vi "Actor Core.vi"(8 "error in":errorcluster, 11 "Square in":refnum<class "Rigol DG822 Pulse.lvclass">) -> (0 "error out":errorcluster, 3 "Actor out":refnum<class "Actor.lvclass">)   [LabVIEW 2021, in "Rigol DG822 UI.lvlib" / "Rigol DG822 Pulse.lvlib" / "Rigol DG822 Pulse.lvclass"]
uses:
  Rigol DG822 Pulse.lvclass
  D:/LabVIEW/General/Files/lvlibp/Actors.lvlibp/Actors/Actors/Actors.lvclass
  General/Files/lvlibp/Actor Framework.lvlibp/1abvi3w/vi.lib/ActorFramework/Actor/Actor.lvclass
  Rigol DG822 UI/lib/controls.llb/FreqUnitHandler.ctl
  Rigol DG822 UI/lib/controls.llb/DataCluster.ctl
  Rigol DG822 UI/lib/controls.llb/PeriodUnitHandler.ctl
  Rigol DG822 UI/lib/controls.llb/AmplUnitHandler.ctl
  Rigol DG822 UI/lib/controls.llb/HighLUnitHandler.ctl
  Rigol DG822 UI/lib/controls.llb/OffsetUnitHandler.ctl
  Rigol DG822 UI/lib/controls.llb/LowLUnitHandler.ctl
  Rigol DG822 UI/lib/controls.llb/FreqUnit.ctl
  Rigol DG822 UI/lib/controls.llb/PeriodUnit.ctl
  Rigol DG822 UI/lib/controls.llb/AmplUnit.ctl
  Rigol DG822 UI/lib/controls.llb/HighLUnit.ctl
  Rigol DG822 UI/lib/controls.llb/OffsetUnit.ctl
  Rigol DG822 UI/lib/controls.llb/LowLUnit.ctl
  Rigol DG822 UI/lib/controls.llb/WaveformParamTags.ctl
  Rigol DG822 UI/lib/controls.llb/PulseParamDisplay.ctl
  Rigol DG822 UI/lib/controls.llb/SliderControl.ctl
  Rigol DG822 UI/lib/controls.llb/PhaseUnitHandler.ctl
  Rigol DG822 UI/lib/controls.llb/DutyUnitHandler.ctl
  Rigol DG822 UI/lib/controls.llb/StringIndicatorSelected.ctl
  Rigol DG822 UI/lib/controls.llb/RDG822ExtCall.ctl
  Rigol DG822 UI/lib/controls.llb/FT Controls Cluster.ctl
  Rigol DG822 Pulse.lvclass/Rigol DG822 Pulse.ctl
  Rigol DG822 UI/lib/controls.llb/WaveformExtCall.ctl
  Rigol DG822 UI/lib/controls.llb/AllWaveformDataCluster.ctl
  Rigol DG822 UI/lib/controls.llb/String Indicators Cluster.ctl
  <vilib>/Utility/miscctls.llb/LVPointTypeDef.ctl
  <userlib>/_MGI/Application Control/MGI VI Reference/MGI Current VI's Reference.vi
  General/Files/lvlibp/Actors.lvlibp/Actors/Actors/Actors.lvclass
panel:
  in  "Slider":T1
  in  "ParamTags":T2
  out "Data":T3={"Freq"={"Freq"=1.0, "FreqUnit"=enum."kHz", "FreqUnitPrcs"=9.0}, "Period"={"Period"=1.0, "PeriodUnit"=enum."ms", "PeriodUnitPrcs"=7.0}, "Ampl"={"Ampl"=5.0, "AmplUnit"=enum."Vpp", "AmplUnitPrcs"=4.0}, "HighL"={"HighL"=2.5, "HighLUnit"=enum."V", "HighLUnitPrcs"=4.0}, "Offset"={"Offset"=0.0, "OffsetUnit"=enum."Vdc", "OffsetUnitPrcs"=4.0}, "LowL"={"LowL"=-2.5, "LowLUnit"=enum."V", "LowLUnitPrcs"=4.0}, "Phase"={"Phase"=0.0, "PhaseUnit"=enum."°", "PhaseUnitPrcs"=3.0}, "Duty"={"Duty"=50.0, "DutyUnit"=enum."%", "DutyUnitPrcs"=3.0}, "Width"={"Width"=500.0, "WidthUnit"=enum."us", "WidthUnitPrcs"=4.0}, "RisEdge"={"RisEdge"=10.0, "RisEdgeUnit"=enum."ns", "RisEdgeUnitPrcs"=1.0}, "FallEdge"={"FallEdge"=10.0, "FallEdgeUnit"=enum."ns", "FallEdgeUnitPrcs"=1.0}} {"RisEdge"."RisEdge" format="%.1f"; "RisEdge"."RisEdgeUnitPrcs" format="%#_1g"; "FallEdge"."FallEdge" format="%.1f"; "FallEdge"."FallEdgeUnitPrcs" format="%#_1g"; "Width"."Width" format="%.4g"; "Width"."WidthUnitPrcs" format="%#_1g"; "Duty"."Duty" format="%.3g"; "Duty"."DutyUnitPrcs" format="%#_1g"; "Phase"."Phase" format="%.3g"; "Phase"."PhaseUnitPrcs" format="%#_1g"; "LowL"."LowL" format="%.4g"; "LowL"."LowLUnitPrcs" format="%#_1g"; "Offset"."Offset" format="%.4g"; "Offset"."OffsetUnitPrcs" format="%#_1g"; "HighL"."HighL" format="%.4g"; "HighL"."HighLUnitPrcs" format="%#_1g"; "Ampl"."Ampl" format="%.4g"; "Ampl"."AmplUnitPrcs" format="%#_1g"; "Period"."Period" format="%.7g"; "Period"."PeriodUnitPrcs" format="%#_1g"; "Freq"."FreqUnitPrcs" format="%#_1g"; "Freq"."Freq" format="%.9g"}
  in  "Conf Tabs":enum32{"Pulse", "OK"}(tab)
  in  "Slider Tab":enum32{"First", "Second"}(tab)
  in  "F/T Ctrls":T4
  out "String Indcs":T5={"Freq-Period"="1.000,000,000 kHz", "Ampl-HighL"="5.000,0 Vpp", "Offset-LowL"="0.000,0 Vdc", "Phase"="0.000 °"}
  in  "F/T Ctrls 2":cluster{"Duty/Width":bool}
  out "String Indcs 2":T6={"Duty-Width"="50.000 %", "RisEdge"="10.0 ns", "FallEdge"="10.0 ns"}
  out "PulseParamDisplay":T7
  in  "Value":dbl=1.0 format="%.8g"
  in  "Unit Tabs":T8(tab)
  out "FreqUnitHandler":T9=1
  in  "FreqUnit":T10=enum."kHz"
  out "PeriodUnitHandler":T11=1
  in  "PeriodUnit":T12=enum."ms"
  in  "AmplUnit":T13=enum."Vpp"
  out "AmplUnitHandler":T14
  out "HighLUnitHandler":T15
  in  "HighLUnit":T16=enum."V"
  out "OffsetUnitHandler":T17
  in  "OffsetUnit":T18=enum."Vdc"
  out "LowLUnitHandler":T19
  in  "LowLUnit":T20=enum."V"
  out "PhaseUnitHandler":T21
  out "DutyUnitHandler":T22
  out "WidthUnitHandler":T11=2
  in  "WidthUnit":T12=enum."us"
  out "RisEdgeUnitHandler":T11=3
  in  "RisEdgeUnit":T12=enum."ns"
  out "FallEdgeUnitHandler":T11=3
  in  "FallEdgeUnit":T12=enum."ns"
  in  "OK":bool
  # "MHz - 10 \nkHz - 9\nHz - 6\nmHz - 3\nuHz - 0"
  # "s - 10\nms - 7\nus - 4 \nns - 1"
  # "All 4 - V - 4\n        mV - 1"
  # "no change"
  # "no change"
  # "s - 10\nms - 7\nus - 4 \nns - 1"
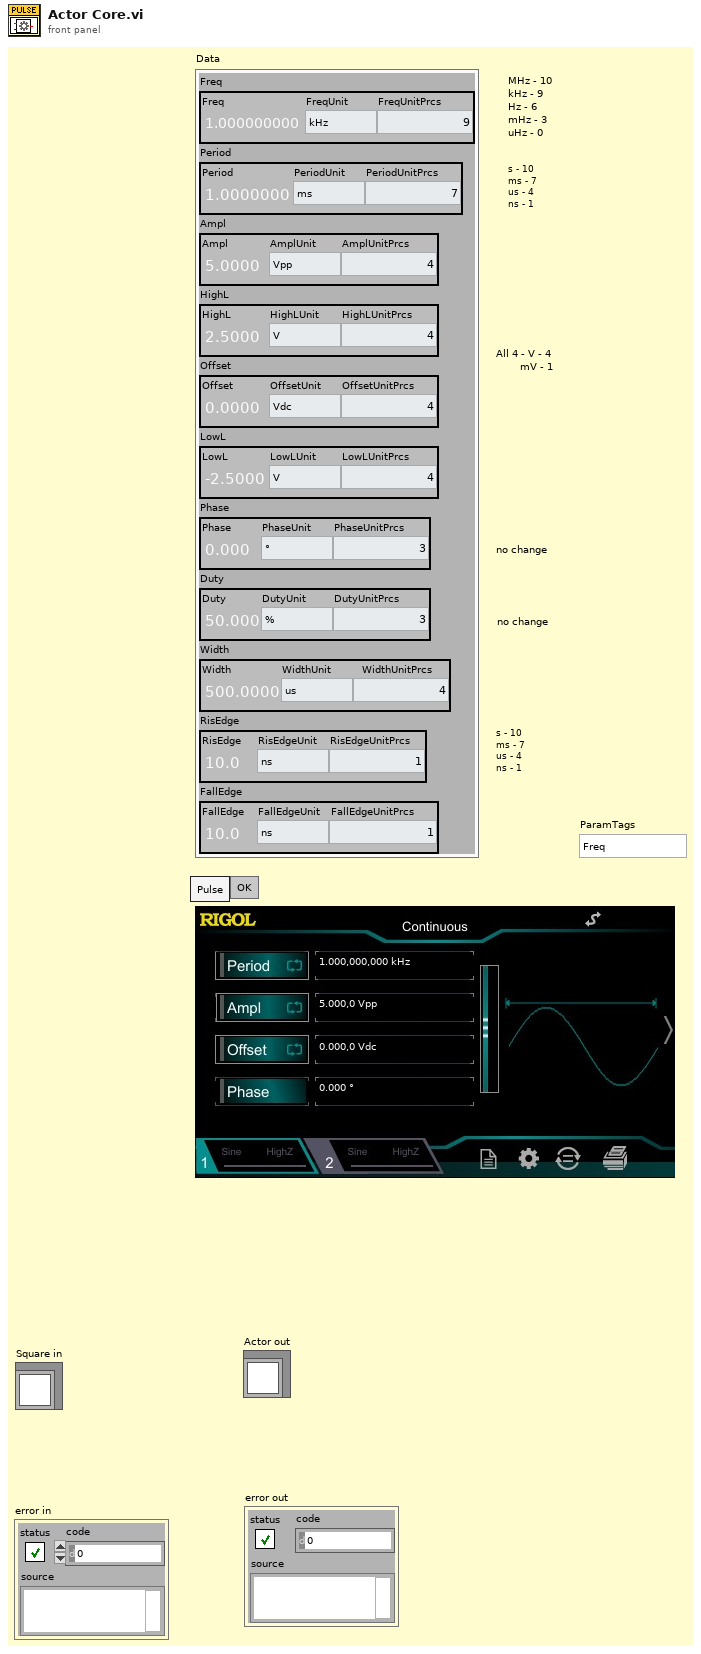
[diagram p1: front panel]
types:
  T1 = typedef "SliderControl.ctl" = bool
  T2 = typedef "WaveformParamTags.ctl" = enum16{"Freq", "Period", "Ampl", "HighL", "Offset", "LowL", "Phase", "Duty", "Width", "RisEdge", "FallEdge"}
  T3 = typedef "DataCluster.ctl" = cluster{"Freq":cluster{"Freq":dbl, "FreqUnit":enum32{"No Selection", "MHz", "kHz", "Hz", "mHz", "uHz"}, "FreqUnitPrcs":dbl}, "Period":cluster{"Period":dbl, "PeriodUnit":enum32{"No Selection", "s", "ms", "us", "ns"}, "PeriodUnitPrcs":dbl}, "Ampl":cluster{"Ampl":dbl, "AmplUnit":enum32{"No Selection", "Vpp", "mVpp"}, "AmplUnitPrcs":dbl}, "HighL":cluster{"HighL":dbl, "HighLUnit":enum32{"No Selection", "V", "mV"}, "HighLUnitPrcs":dbl}, "Offset":cluster{"Offset":dbl, "OffsetUnit":enum32{"No Selection", "Vdc", "mVdc"}, "OffsetUnitPrcs":dbl}, "LowL":cluster{"LowL":dbl, "LowLUnit":enum32{"No Selection", "V", "mV"}, "LowLUnitPrcs":dbl}, "Phase":cluster{"Phase":dbl, "PhaseUnit":enum32{"°"}, "PhaseUnitPrcs":dbl}, "Duty":cluster{"Duty":dbl, "DutyUnit":enum32{"%"}, "DutyUnitPrcs":dbl}, "Width":cluster{"Width":dbl, "WidthUnit":enum32{"No Selection", "s", "ms", "us", "ns"}, "WidthUnitPrcs":dbl}, "RisEdge":cluster{"RisEdge":dbl, "RisEdgeUnit":enum32{"No Selection", "s", "ms", "us", "ns"}, "RisEdgeUnitPrcs":dbl}, "FallEdge":cluster{"FallEdge":dbl, "FallEdgeUnit":enum32{"No Selection", "s", "ms", "us", "ns"}, "FallEdgeUnitPrcs":dbl}}
  T4 = cluster{"Freq/Period":bool, "Ampl/HighL":bool, "Offset/LowL":bool}
  T5 = cluster{"Freq-Period":string, "Ampl-HighL":string, "Offset-LowL":string, "Phase":string}
  T6 = cluster{"Duty-Width":string, "RisEdge":string, "FallEdge":string}
  T7 = typedef "PulseParamDisplay.ctl" = u16
  T8 = enum32{"Freq", "Period", "Ampl", "HighL", "Offset", "LowL", "Phase", "Duty", "Width", "RisEdge", "FallEdge"}
  T9 = typedef "FreqUnitHandler.ctl" = u16
  T10 = typedef "FreqUnit.ctl" = enum32{"No Selection", "MHz", "kHz", "Hz", "mHz", "uHz"}
  T11 = typedef "PeriodUnitHandler.ctl" = u16
  T12 = typedef "PeriodUnit.ctl" = enum32{"No Selection", "s", "ms", "us", "ns"}
  T13 = typedef "AmplUnit.ctl" = enum32{"No Selection", "Vpp", "mVpp"}
  T14 = typedef "AmplUnitHandler.ctl" = u16
  T15 = typedef "HighLUnitHandler.ctl" = u16
  T16 = typedef "HighLUnit.ctl" = enum32{"No Selection", "V", "mV"}
  T17 = typedef "OffsetUnitHandler.ctl" = u16
  T18 = typedef "OffsetUnit.ctl" = enum32{"No Selection", "Vdc", "mVdc"}
  T19 = typedef "LowLUnitHandler.ctl" = u16
  T20 = typedef "LowLUnit.ctl" = enum32{"No Selection", "V", "mV"}
  T21 = typedef "PhaseUnitHandler.ctl" = u16
  T22 = typedef "DutyUnitHandler.ctl" = u16
  T23 = cluster{"Freq-Period":string, "Freq-Period 2":string, "Freq-Period 3":string, "Freq-Period 4":string, "Freq-Period 5":string, "Freq-Period 6":string, "Freq-Period 7":string}
  T24 = typedef "LVPointTypeDef.ctl" = cluster{"Horizontal":i16, "Vertical":i16}
  T25 = typedef "StringIndicatorSelected.ctl" = enum16{"Freq-Period", "Ampl-HighL", "Offset-LowL", "Phase", "Duty-Width", "RisEdge", "FallEdge"}
  T26 = typedef "FT Controls Cluster.ctl" = cluster{"Freq/Period":bool, "Ampl/HighL":bool, "Offset/LowL":bool, "Duty/Width":bool}
  T27 = typedef "RDG822ExtCall.ctl" = enum16{"Get Data"}
  T28 = typedef "WaveformExtCall.ctl" = enum16{"Freq", "Period", "Ampl", "HighL", "Offset", "LowL", "Phase", "Duty", "Width", "RisEdge", "FallEdge", "Home", "InitData"}
  T29 = cluster{"Freq":cluster{"Freq":dbl, "FreqUnit":enum32{"No Selection", "MHz", "kHz", "Hz", "mHz", "uHz"}, "FreqUnitPrcs":dbl}, "Period":cluster{"Period":dbl, "PeriodUnit":enum32{"No Selection", "s", "ms", "us", "ns"}, "PeriodUnitPrcs":dbl}, "Duty":cluster{"Duty":dbl, "DutyUnit":enum32{"%"}, "DutyUnitPrcs":dbl}, "Width":cluster{"Width":dbl, "WidthUnit":enum32{"No Selection", "s", "ms", "us", "ns"}, "WidthUnitPrcs":dbl}, "RisEdge":cluster{"RisEdge":dbl, "RisEdgeUnit":enum32{"No Selection", "s", "ms", "us", "ns"}, "RisEdgeUnitPrcs":dbl}, "FallEdge":cluster{"FallEdge":dbl, "FallEdgeUnit":enum32{"No Selection", "s", "ms", "us", "ns"}, "FallEdgeUnitPrcs":dbl}}
  T30 = cluster{"Ampl":cluster{"Ampl":dbl, "AmplUnit":enum32{"No Selection", "Vpp", "mVpp"}, "AmplUnitPrcs":dbl}, "HighL":cluster{"HighL":dbl, "HighLUnit":enum32{"No Selection", "V", "mV"}, "HighLUnitPrcs":dbl}, "Offset":cluster{"Offset":dbl, "OffsetUnit":enum32{"No Selection", "Vdc", "mVdc"}, "OffsetUnitPrcs":dbl}, "LowL":cluster{"LowL":dbl, "LowLUnit":enum32{"No Selection", "V", "mV"}, "LowLUnitPrcs":dbl}}
  T31 = cluster{"Phase":dbl, "PhaseUnit":enum32{"°"}, "PhaseUnitPrcs":dbl}
  T32 = cluster{"Duty":cluster{"Duty":dbl, "DutyUnit":enum32{"%"}, "DutyUnitPrcs":dbl}, "Width":cluster{"Width":dbl, "WidthUnit":enum32{"No Selection", "s", "ms", "us", "ns"}, "WidthUnitPrcs":dbl}, "FallEdge":cluster{"FallEdge":dbl, "FallEdgeUnit":enum32{"No Selection", "s", "ms", "us", "ns"}, "FallEdgeUnitPrcs":dbl}, "RisEdge":cluster{"RisEdge":dbl, "RisEdgeUnit":enum32{"No Selection", "s", "ms", "us", "ns"}, "RisEdgeUnitPrcs":dbl}}
  T33 = cluster{"FallEdge":cluster{"FallEdge":dbl, "FallEdgeUnit":enum32{"No Selection", "s", "ms", "us", "ns"}, "FallEdgeUnitPrcs":dbl}, "RisEdge":cluster{"RisEdge":dbl, "RisEdgeUnit":enum32{"No Selection", "s", "ms", "us", "ns"}, "RisEdgeUnitPrcs":dbl}}
  T34 = typedef "AllWaveformDataCluster.ctl" = cluster{"Data":T3, "F/T Ctrls":T26, "String Indcs":T35}
  T35 = typedef "String Indicators Cluster.ctl" = cluster{"Freq-Period":string, "Ampl-HighL":string, "Offset-LowL":string, "Phase":string, "Duty-Width":string, "RisEdge":string, "FallEdge":string}
  T36 = cluster{"Freq/Period":bool, "Ampl/HighL":bool, "Offset/LowL":bool, "Duty/Width":bool}
  T37 = enum32{"No Selection", "MHz", "kHz", "Hz", "mHz", "uHz"}
  T38 = cluster{"Value":dbl, "PeriodUnit":u32, "FreqUnitPrecision":dbl}
  T39 = cluster{"Freq":dbl, "FreqUnit":enum32{"No Selection", "MHz", "kHz", "Hz", "mHz", "uHz"}, "FreqUnitPrcs":dbl}
  T40 = cluster{"Period":dbl, "PeriodUnit":enum32{"No Selection", "s", "ms", "us", "ns"}, "PeriodUnitPrcs":dbl}
  T41 = cluster{"Duty":dbl, "DutyUnit":enum32{"%"}, "DutyUnitPrcs":dbl}
  T42 = cluster{"Width":dbl, "WidthUnit":enum32{"No Selection", "s", "ms", "us", "ns"}, "WidthUnitPrcs":dbl}
  T43 = cluster{"RisEdge":dbl, "RisEdgeUnit":enum32{"No Selection", "s", "ms", "us", "ns"}, "RisEdgeUnitPrcs":dbl}
  T44 = cluster{"FallEdge":dbl, "FallEdgeUnit":enum32{"No Selection", "s", "ms", "us", "ns"}, "FallEdgeUnitPrcs":dbl}
  T45 = cluster{"Ampl":dbl, "AmplUnit":enum32{"No Selection", "Vpp", "mVpp"}, "AmplUnitPrcs":dbl}
  T46 = cluster{"HighL":dbl, "HighLUnit":enum32{"No Selection", "V", "mV"}, "HighLUnitPrcs":dbl}
  T47 = cluster{"Offset":dbl, "OffsetUnit":enum32{"No Selection", "Vdc", "mVdc"}, "OffsetUnitPrcs":dbl}
  T48 = cluster{"LowL":dbl, "LowLUnit":enum32{"No Selection", "V", "mV"}, "LowLUnitPrcs":dbl}
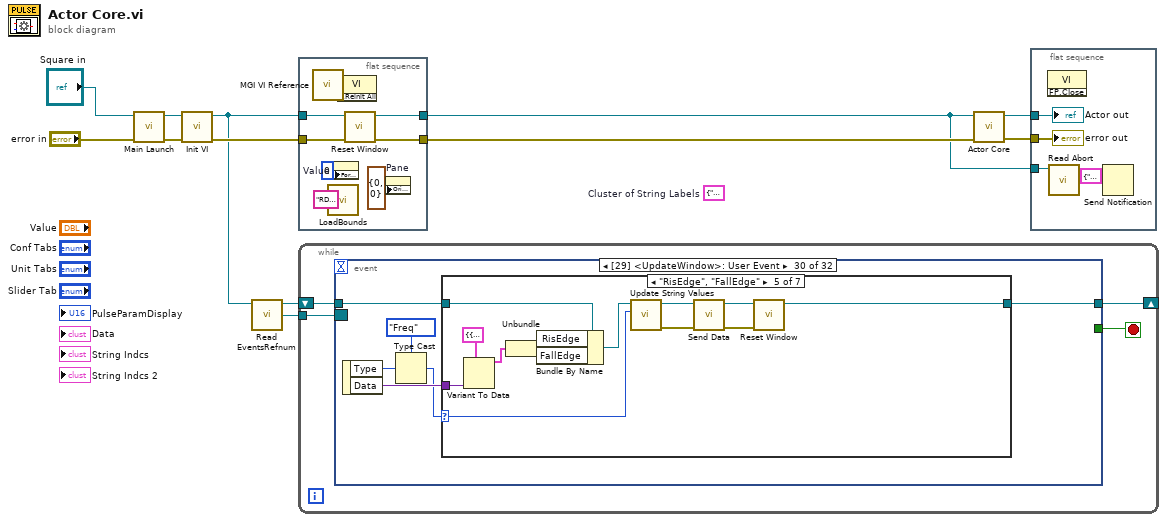
[diagram p0: block diagram]
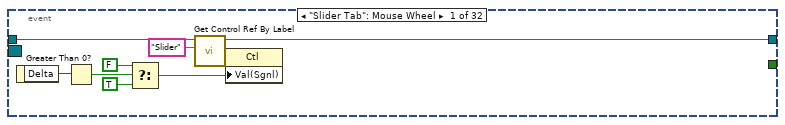
[diagram p2: hidden frame]
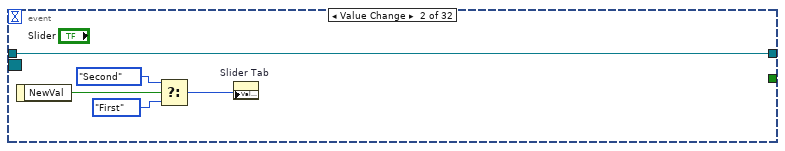
[diagram p3: hidden frame]
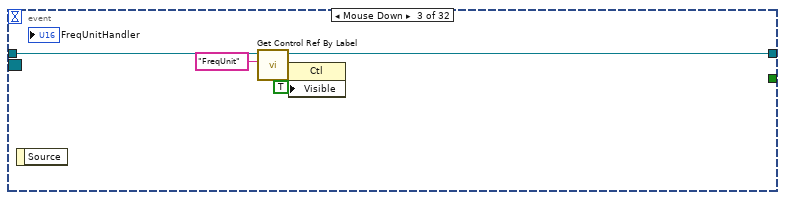
[diagram p4: hidden frame]
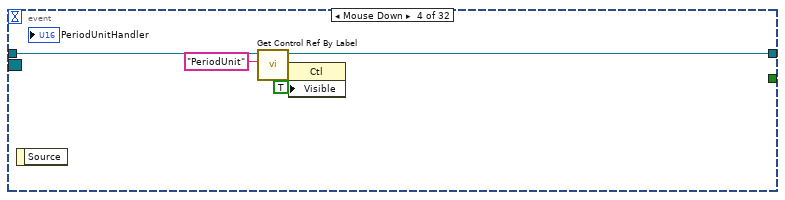
[diagram p5: hidden frame]
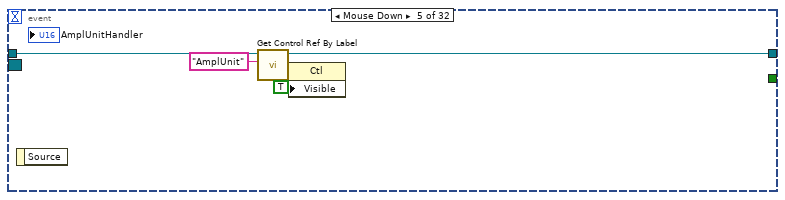
[diagram p6: hidden frame]
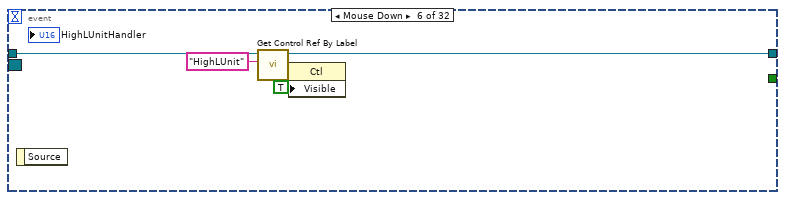
[diagram p7: hidden frame]
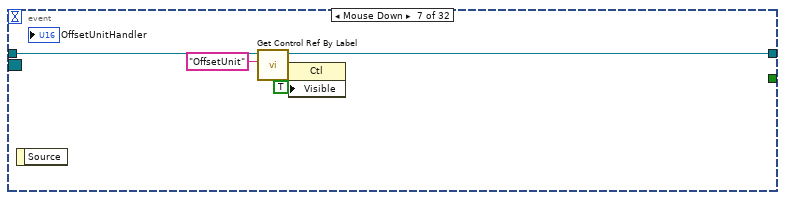
[diagram p8: hidden frame]
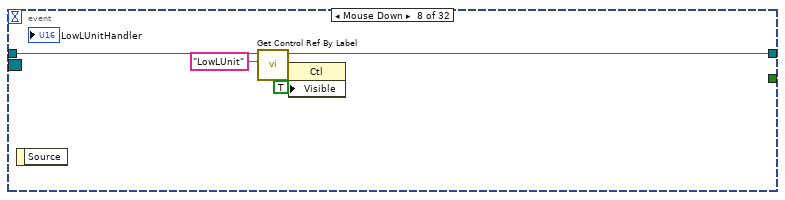
[diagram p9: hidden frame]
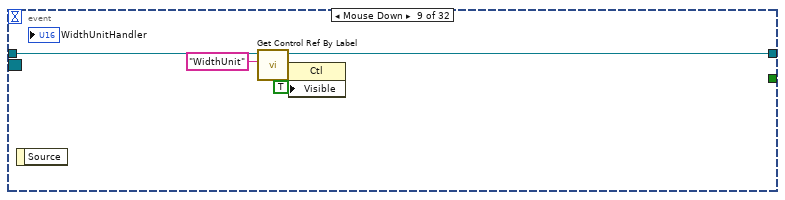
[diagram p10: hidden frame]
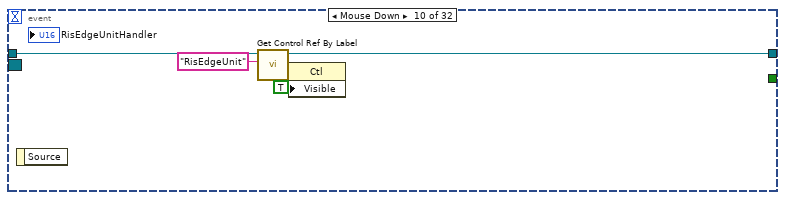
[diagram p11: hidden frame]
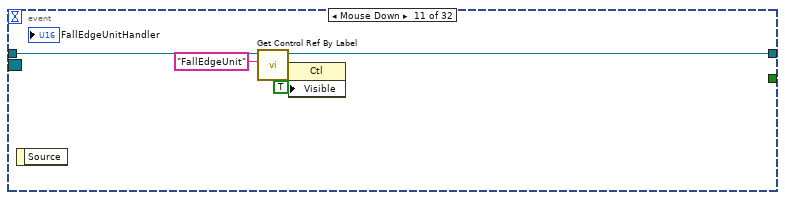
[diagram p12: hidden frame]
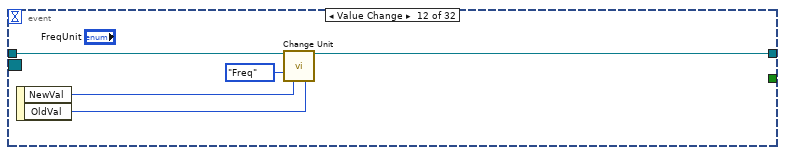
[diagram p13: hidden frame]
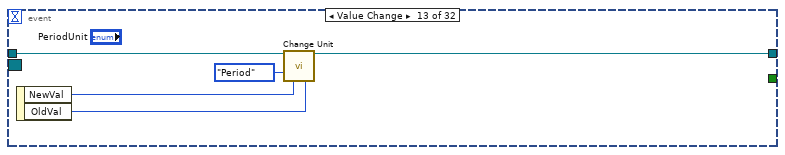
[diagram p14: hidden frame]
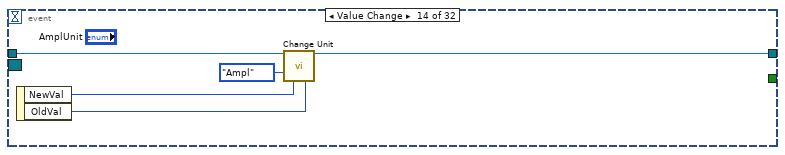
[diagram p15: hidden frame]
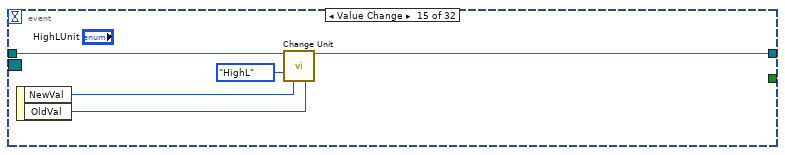
[diagram p16: hidden frame]
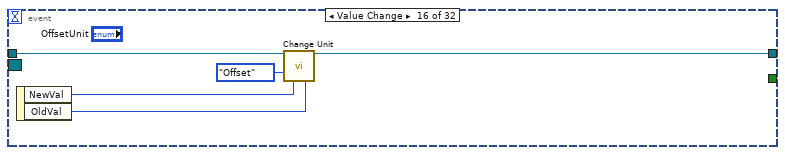
[diagram p17: hidden frame]
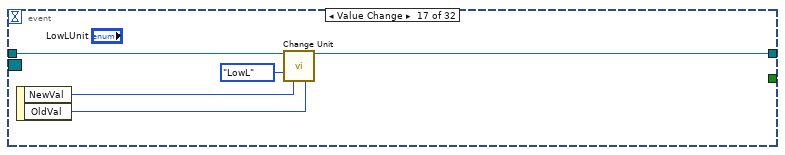
[diagram p18: hidden frame]
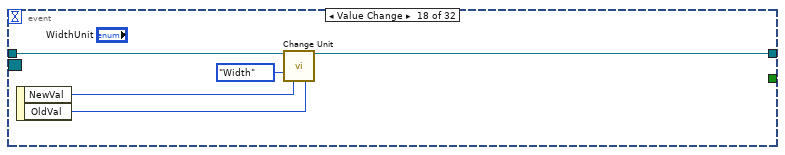
[diagram p19: hidden frame]
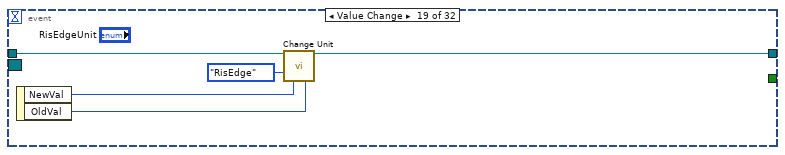
[diagram p20: hidden frame]
diagram:
  (unwired) T23 {"Freq-Period"="String Indcs.Freq-Period", "Freq-Period 2"="String Indcs.Ampl-HighL", "Freq-Period 3"="String Indcs.Offset-LowL", "Freq-Period 4"="String Indcs.Phase", "Freq-Period 5"="String Indcs 2.Duty-Width", "Freq-Period 6"="String Indcs 2.RisEdge", "Freq-Period 7"="String Indcs 2.Falldge"}  # Cluster of String Labels
  n1 = call "Main Launch.vi"("error in (no error)"="error in", "Actors in"="Square in") -> ("error out"=w4:errorcluster, "Actors out"=w3:refnum<class "Rigol DG822 Pulse.lvclass">)  [unwired: 6 in, 2 out]
  n2 = call-dynamic "Init VI.vi"("error in (no error)"=w4, "Rigol DG822 Pulse in"=w3) -> ("error out"=w5:errorcluster, "Rigol DG822 Pulse out"=w2:refnum<class "Rigol DG822 Pulse.lvclass">)  [unwired: 8 in]
  n3 = call "Read EventsRefnum.vi"("Actors in"=w2) -> ("EventsRefnum"=w8:refnum<event-registration>, "Actors out"=w7:refnum<class "Rigol DG822 Pulse.lvclass">)  [unwired: 9 in]
  n4 = flat-sequence {
    tunnel: w5 -> [w15]
    tunnel: [w18] -> w10
    tunnel: w2 -> [w16]
    tunnel: [w17] -> w6
    frame #0 {
      n5 = call-poly <userlib>:"MGI VI Reference.vi"() -> ("Current VI's Reference"=w14:refnum<vi>)  [unwired: 1 in]
      n6 = call "LoadBounds.vi"("SettingName"="RDG822Pulse.bounds") -> ()
      n7 = property on="Value" class="DigNum (strict)"("Format"=u8 0 ("Display Format:Format")) -> ()  [unwired: 2 in, 2 out]
      n8 = invoke class="VI" method="Default Vals.Reinit All"(reference=w14) -> ()  [unwired: 2 in, 3 out]
      n9 = call-dynamic "Reset Window.vi"("error in (no error)"=w15, "Rigol DG822 Pulse in"=w16) -> ("error out"=w18:errorcluster, "Rigol DG822 Pulse out"=w17:refnum<class "Rigol DG822 Pulse.lvclass">)  [unwired: 8 in]
      n10 = property on="Pane" class="Pane"("Origin"=T24 {"Horizontal"=0, "Vertical"=0}) -> ()  [unwired: 2 in, 2 out]
    }
  }
  n11 = while {
    tunnel: w8 -> [w24]
    shift-right: [w22] -> _
    shift-left: w7 -> [w23]
    stop <- w21 stop-if-true
    n12 = event shown="[29] <UpdateWindow>: User Event" {
      selector: w24 -> [_ _ _ _ _ _ _ _ _ _ _ _ _ _ _ _ _ _ _ _ _ _ _ _ _ _ _ _ _ _ _ w370]
      dyn-events: _ -> [_ _ _ _ _ _ _ _ _ _ _ _ _ _ _ _ _ _ _ _ _ _ _ _ _ _ _ _ _ _ _ _]
      timeout: _ -> [_ _ _ _ _ _ _ _ _ _ _ _ _ _ _ _ _ _ _ _ _ _ _ _ _ _ _ _ _ _ _ _]
      tunnel: w23 -> [w25 w39 w45 w51 w57 w63 w69 w75 w81 w87 w93 w98 w103 w108 w113 w118 w123 w128 w133 w138 w140 w147 w152 w157 w162 w167 w172 w183 w203 w247 w358 w368]
      tunnel: [w26 w39 w44 w50 w56 w62 w68 w74 w80 w86 w92 w97 w102 w107 w112 w117 w122 w127 w132 w137 w143 w148 w153 w158 w163 w168 w173 w184 w197 w248 w355 w366] -> w22
      tunnel: [_ _ _ _ _ _ _ _ _ _ _ _ _ _ _ _ _ _ _ _ _ _ _ _ _ _ _ _ _ _ _ w371] -> w21
      event "Slider Tab": Mouse Wheel {
        n13 = event-data() -> ("Delta"=w34:i32)  [unwired: 1 in]
        n14 = Greater Than 0?(x=w34) -> (x > 0?=w33:bool)
        n15 = Select(t=FALSE, s=w33, f=TRUE) -> (s? t:f=w27:bool)
        n16 = call "Get Control Ref By Label.vi"("Control Label"="Slider", "Actors in"=w25) -> ("error out"=w29:errorcluster, "Control Ref"=w30:refnum<vi>, "Actors out"=w26:refnum<class "Rigol DG822 Pulse.lvclass">)  [unwired: 7 in]
        n17 = property class="Ctl"(reference=w30, error in=w29, "Val(Sgnl)"=w27) -> ()  [unwired: 2 out]
      }
      event Value Change {
        n18 = event-data() -> ("NewVal"=w35:T1)  [unwired: 1 in]
        n19 = Select(t=enum32{"First", "Second"}."Second" ("Slider Tab"), s=w35, f=enum32{"First", "Second"}."First" ("Slider Tab")) -> (s? t:f=w36:enum32{"First", "Second"})
        n20 = property on="Slider Tab" class="TabCtl (strict)"("Value"=w36) -> ()  [unwired: 2 in, 2 out]
      }
      event Mouse Down {
        n21 = event-data() -> ()  [unwired: 1 in, 1 out]
        n22 = call "Get Control Ref By Label.vi"("Control Label"="FreqUnit", "Actors in"=w45) -> ("error out"=w40:errorcluster, "Control Ref"=w42:refnum<vi>, "Actors out"=w44:refnum<class "Rigol DG822 Pulse.lvclass">)  [unwired: 7 in]
        n23 = property class="Ctl"(reference=w42, error in=w40, "Visible"=TRUE) -> ()  [unwired: 2 out]
      }
      event Mouse Down {
        n24 = event-data() -> ()  [unwired: 1 in, 1 out]
        n25 = call "Get Control Ref By Label.vi"("Control Label"="PeriodUnit", "Actors in"=w51) -> ("error out"=w46:errorcluster, "Control Ref"=w48:refnum<vi>, "Actors out"=w50:refnum<class "Rigol DG822 Pulse.lvclass">)  [unwired: 7 in]
        n26 = property class="Ctl"(reference=w48, error in=w46, "Visible"=TRUE) -> ()  [unwired: 2 out]
      }
      event Mouse Down {
        n27 = event-data() -> ()  [unwired: 1 in, 1 out]
        n28 = call "Get Control Ref By Label.vi"("Control Label"="AmplUnit", "Actors in"=w57) -> ("error out"=w52:errorcluster, "Control Ref"=w54:refnum<vi>, "Actors out"=w56:refnum<class "Rigol DG822 Pulse.lvclass">)  [unwired: 7 in]
        n29 = property class="Ctl"(reference=w54, error in=w52, "Visible"=TRUE) -> ()  [unwired: 2 out]
      }
      event Mouse Down {
        n30 = event-data() -> ()  [unwired: 1 in, 1 out]
        n31 = call "Get Control Ref By Label.vi"("Control Label"="HighLUnit", "Actors in"=w63) -> ("error out"=w58:errorcluster, "Control Ref"=w60:refnum<vi>, "Actors out"=w62:refnum<class "Rigol DG822 Pulse.lvclass">)  [unwired: 7 in]
        n32 = property class="Ctl"(reference=w60, error in=w58, "Visible"=TRUE) -> ()  [unwired: 2 out]
      }
      event Mouse Down {
        n33 = event-data() -> ()  [unwired: 1 in, 1 out]
        n34 = call "Get Control Ref By Label.vi"("Control Label"="OffsetUnit", "Actors in"=w69) -> ("error out"=w64:errorcluster, "Control Ref"=w66:refnum<vi>, "Actors out"=w68:refnum<class "Rigol DG822 Pulse.lvclass">)  [unwired: 7 in]
        n35 = property class="Ctl"(reference=w66, error in=w64, "Visible"=TRUE) -> ()  [unwired: 2 out]
      }
      event Mouse Down {
        n36 = event-data() -> ()  [unwired: 1 in, 1 out]
        n37 = call "Get Control Ref By Label.vi"("Control Label"="LowLUnit", "Actors in"=w75) -> ("error out"=w70:errorcluster, "Control Ref"=w72:refnum<vi>, "Actors out"=w74:refnum<class "Rigol DG822 Pulse.lvclass">)  [unwired: 7 in]
        n38 = property class="Ctl"(reference=w72, error in=w70, "Visible"=TRUE) -> ()  [unwired: 2 out]
      }
      event Mouse Down {
        n39 = event-data() -> ()  [unwired: 1 in, 1 out]
        n40 = call "Get Control Ref By Label.vi"("Control Label"="WidthUnit", "Actors in"=w81) -> ("error out"=w76:errorcluster, "Control Ref"=w78:refnum<vi>, "Actors out"=w80:refnum<class "Rigol DG822 Pulse.lvclass">)  [unwired: 7 in]
        n41 = property class="Ctl"(reference=w78, error in=w76, "Visible"=TRUE) -> ()  [unwired: 2 out]
      }
      event Mouse Down {
        n42 = event-data() -> ()  [unwired: 1 in, 1 out]
        n43 = call "Get Control Ref By Label.vi"("Control Label"="RisEdgeUnit", "Actors in"=w87) -> ("error out"=w82:errorcluster, "Control Ref"=w84:refnum<vi>, "Actors out"=w86:refnum<class "Rigol DG822 Pulse.lvclass">)  [unwired: 7 in]
        n44 = property class="Ctl"(reference=w84, error in=w82, "Visible"=TRUE) -> ()  [unwired: 2 out]
      }
      event Mouse Down {
        n45 = event-data() -> ()  [unwired: 1 in, 1 out]
        n46 = call "Get Control Ref By Label.vi"("Control Label"="FallEdgeUnit", "Actors in"=w93) -> ("error out"=w88:errorcluster, "Control Ref"=w90:refnum<vi>, "Actors out"=w92:refnum<class "Rigol DG822 Pulse.lvclass">)  [unwired: 7 in]
        n47 = property class="Ctl"(reference=w90, error in=w88, "Visible"=TRUE) -> ()  [unwired: 2 out]
      }
      event Value Change {
        n48 = event-data() -> ("NewVal"=w96:T10, "OldVal"=w95:T10)  [unwired: 1 in]
        n49 = call-dynamic "Change Unit.vi"("Rigol DG822 Pulse in"=w98, "ParamTags"=WaveformParamTags."Freq", "New Value"=w96, "Old Value"=w95) -> ("Rigol DG822 Pulse out"=w97:refnum<class "Rigol DG822 Pulse.lvclass">)  [unwired: 10 in, 1 out]
      }
      event Value Change {
        n50 = event-data() -> ("NewVal"=w101:T12, "OldVal"=w100:T12)  [unwired: 1 in]
        n51 = call-dynamic "Change Unit.vi"("Rigol DG822 Pulse in"=w103, "ParamTags"=WaveformParamTags."Period", "New Value"=w101, "Old Value"=w100) -> ("Rigol DG822 Pulse out"=w102:refnum<class "Rigol DG822 Pulse.lvclass">)  [unwired: 10 in, 1 out]
      }
      event Value Change {
        n52 = event-data() -> ("NewVal"=w106:T13, "OldVal"=w105:T13)  [unwired: 1 in]
        n53 = call-dynamic "Change Unit.vi"("Rigol DG822 Pulse in"=w108, "ParamTags"=WaveformParamTags."Ampl", "New Value"=w106, "Old Value"=w105) -> ("Rigol DG822 Pulse out"=w107:refnum<class "Rigol DG822 Pulse.lvclass">)  [unwired: 10 in, 1 out]
      }
      event Value Change {
        n54 = event-data() -> ("NewVal"=w111:T16, "OldVal"=w110:T16)  [unwired: 1 in]
        n55 = call-dynamic "Change Unit.vi"("Rigol DG822 Pulse in"=w113, "ParamTags"=WaveformParamTags."HighL", "New Value"=w111, "Old Value"=w110) -> ("Rigol DG822 Pulse out"=w112:refnum<class "Rigol DG822 Pulse.lvclass">)  [unwired: 10 in, 1 out]
      }
      event Value Change {
        n56 = event-data() -> ("NewVal"=w116:T18, "OldVal"=w115:T18)  [unwired: 1 in]
        n57 = call-dynamic "Change Unit.vi"("Rigol DG822 Pulse in"=w118, "ParamTags"=WaveformParamTags."Offset", "New Value"=w116, "Old Value"=w115) -> ("Rigol DG822 Pulse out"=w117:refnum<class "Rigol DG822 Pulse.lvclass">)  [unwired: 10 in, 1 out]
      }
      event Value Change {
        n58 = event-data() -> ("NewVal"=w121:T20, "OldVal"=w120:T20)  [unwired: 1 in]
        n59 = call-dynamic "Change Unit.vi"("Rigol DG822 Pulse in"=w123, "ParamTags"=WaveformParamTags."LowL", "New Value"=w121, "Old Value"=w120) -> ("Rigol DG822 Pulse out"=w122:refnum<class "Rigol DG822 Pulse.lvclass">)  [unwired: 10 in, 1 out]
      }
      event Value Change {
        n60 = event-data() -> ("NewVal"=w126:T12, "OldVal"=w125:T12)  [unwired: 1 in]
        n61 = call-dynamic "Change Unit.vi"("Rigol DG822 Pulse in"=w128, "ParamTags"=WaveformParamTags."Width", "New Value"=w126, "Old Value"=w125) -> ("Rigol DG822 Pulse out"=w127:refnum<class "Rigol DG822 Pulse.lvclass">)  [unwired: 10 in, 1 out]
      }
      event Value Change {
        n62 = event-data() -> ("NewVal"=w131:T12, "OldVal"=w130:T12)  [unwired: 1 in]
        n63 = call-dynamic "Change Unit.vi"("Rigol DG822 Pulse in"=w133, "ParamTags"=WaveformParamTags."RisEdge", "New Value"=w131, "Old Value"=w130) -> ("Rigol DG822 Pulse out"=w132:refnum<class "Rigol DG822 Pulse.lvclass">)  [unwired: 10 in, 1 out]
      }
      event Value Change {
        n64 = event-data() -> ("NewVal"=w136:T12, "OldVal"=w135:T12)  [unwired: 1 in]
        n65 = call-dynamic "Change Unit.vi"("Rigol DG822 Pulse in"=w138, "ParamTags"=WaveformParamTags."FallEdge", "New Value"=w136, "Old Value"=w135) -> ("Rigol DG822 Pulse out"=w137:refnum<class "Rigol DG822 Pulse.lvclass">)  [unwired: 10 in, 1 out]
      }
      event "String Indcs.Freq-Period": Mouse Down {
        n66 = event-data() -> ()  [unwired: 1 in, 2 out]
        n67 = call-dynamic "Config OK Tab.vi"("String Selected"=StringIndicatorSelected."Freq-Period", "Rigol DG822 Pulse in"=w140) -> ("error out"=w142:errorcluster, "Rigol DG822 Pulse out"=w143:refnum<class "Rigol DG822 Pulse.lvclass">)  [unwired: 8 in]
        n68 = property on="Conf Tabs" class="TabCtl (strict)"(error in=w142, "Value"=enum32{"Pulse", "OK"}."OK" ("Conf Tabs")) -> ()  [unwired: 1 in, 2 out]
      }
      event "String Indcs.Ampl-HighL": Mouse Down {
        n69 = event-data() -> ()  [unwired: 1 in, 2 out]
        n70 = call-dynamic "Config OK Tab.vi"("String Selected"=StringIndicatorSelected."Ampl-HighL", "Rigol DG822 Pulse in"=w147) -> ("error out"=w146:errorcluster, "Rigol DG822 Pulse out"=w148:refnum<class "Rigol DG822 Pulse.lvclass">)  [unwired: 8 in]
        n71 = property on="Conf Tabs" class="TabCtl (strict)"(error in=w146, "Value"=enum32{"Pulse", "OK"}."OK" ("Conf Tabs")) -> ()  [unwired: 1 in, 2 out]
      }
      event "String Indcs.Offset-LowL": Mouse Down {
        n72 = event-data() -> ()  [unwired: 1 in, 2 out]
        n73 = call-dynamic "Config OK Tab.vi"("String Selected"=StringIndicatorSelected."Offset-LowL", "Rigol DG822 Pulse in"=w152) -> ("error out"=w151:errorcluster, "Rigol DG822 Pulse out"=w153:refnum<class "Rigol DG822 Pulse.lvclass">)  [unwired: 8 in]
        n74 = property on="Conf Tabs" class="TabCtl (strict)"(error in=w151, "Value"=enum32{"Pulse", "OK"}."OK" ("Conf Tabs")) -> ()  [unwired: 1 in, 2 out]
      }
      event "String Indcs.Phase": Mouse Down {
        n75 = event-data() -> ()  [unwired: 1 in, 2 out]
        n76 = call-dynamic "Config OK Tab.vi"("String Selected"=StringIndicatorSelected."Phase", "Rigol DG822 Pulse in"=w157) -> ("error out"=w156:errorcluster, "Rigol DG822 Pulse out"=w158:refnum<class "Rigol DG822 Pulse.lvclass">)  [unwired: 8 in]
        n77 = property on="Conf Tabs" class="TabCtl (strict)"(error in=w156, "Value"=enum32{"Pulse", "OK"}."OK" ("Conf Tabs")) -> ()  [unwired: 1 in, 2 out]
      }
      event "String Indcs 2.Duty-Width": Mouse Down {
        n78 = event-data() -> ()  [unwired: 1 in, 2 out]
        n79 = call-dynamic "Config OK Tab.vi"("String Selected"=StringIndicatorSelected."Duty-Width", "Rigol DG822 Pulse in"=w162) -> ("error out"=w161:errorcluster, "Rigol DG822 Pulse out"=w163:refnum<class "Rigol DG822 Pulse.lvclass">)  [unwired: 8 in]
        n80 = property on="Conf Tabs" class="TabCtl (strict)"(error in=w161, "Value"=enum32{"Pulse", "OK"}."OK" ("Conf Tabs")) -> ()  [unwired: 1 in, 2 out]
      }
      event "String Indcs 2.RisEdge": Mouse Down {
        n81 = event-data() -> ()  [unwired: 1 in, 2 out]
        n82 = call-dynamic "Config OK Tab.vi"("String Selected"=StringIndicatorSelected."RisEdge", "Rigol DG822 Pulse in"=w167) -> ("error out"=w166:errorcluster, "Rigol DG822 Pulse out"=w168:refnum<class "Rigol DG822 Pulse.lvclass">)  [unwired: 8 in]
        n83 = property on="Conf Tabs" class="TabCtl (strict)"(error in=w166, "Value"=enum32{"Pulse", "OK"}."OK" ("Conf Tabs")) -> ()  [unwired: 1 in, 2 out]
      }
      event "String Indcs 2.FallEdge": Mouse Down {
        n84 = event-data() -> ()  [unwired: 1 in, 2 out]
        n85 = call-dynamic "Config OK Tab.vi"("String Selected"=StringIndicatorSelected."FallEdge", "Rigol DG822 Pulse in"=w172) -> ("error out"=w171:errorcluster, "Rigol DG822 Pulse out"=w173:refnum<class "Rigol DG822 Pulse.lvclass">)  [unwired: 8 in]
        n86 = property on="Conf Tabs" class="TabCtl (strict)"(error in=w171, "Value"=enum32{"Pulse", "OK"}."OK" ("Conf Tabs")) -> ()  [unwired: 1 in, 2 out]
      }
      event "F/T Ctrls", "F/T Ctrls 2": Value Change {
        n87 = event-data() -> ()  [unwired: 1 in, 1 out]
        n88 = Unbundle("F/T Ctrls") -> ("Freq/Period"=w177:bool, "Ampl/HighL"=w178:bool, "Offset/LowL"=w179:bool)
        n89 = Unbundle("F/T Ctrls 2") -> ("Duty/Width"=w180:bool)
        n90 = Bundle("Freq/Period"=w177, "Ampl/HighL"=w178, "Offset/LowL"=w179, "Duty/Width"=w180) -> (w182:T36)  [unwired: 1 in]
        n91 = To Variant(anything=w182) -> (Variant=w175:variant)
        n92 = call-dynamic "FT Controls Change.vi"("F/T Controls Cluster Variant"=w175, "Rigol DG822 Pulse in"=w183) -> ("error out"=w187:errorcluster, "New F/T Controls Cluster Variant"=w191:variant, "Rigol DG822 Pulse out"=w192:refnum<class "Rigol DG822 Pulse.lvclass">)  [unwired: 7 in]
        n93 = Variant To Data(error in=w187, type=T26 {"Freq/Period"=FALSE, "Ampl/HighL"=FALSE, "Offset/LowL"=FALSE, "Duty/Width"=FALSE} ("F/T Ctrls"), Variant=w191) -> (data=w190:T26, error out=w174:errorcluster)
        n94 = Bundle By Name(cluster=w192, "F/T Ctrls"=w190) -> (w184:refnum<class "Rigol DG822 Pulse.lvclass">)
        n95 = Unbundle By Name(w184) -> ("RDG822 UI Enq"=w189:refnum<class "Message Enqueuer.lvclass">, "Params Data"=w188:T34)
        n96 = call "Send ExtCall.vi"("error in (no error)"=w174, "Val"=w188, "Tag"=RDG822ExtCall."Get Data", "Message Enqueuer"=w189) -> ()  [unwired: 4 in, 4 out]
      }
      event "OK": Value Change {
        n97 = event-data() -> ()  [unwired: 1 in, 2 out]
        n98 = case shown="\"FallEdge\"" "ParamTags" {
          tunnel: [w209 w212 w215 w218 w221 w224 w227 w230 w233 w236 w239 4.0 ("FreqUnitPrecision")] -> w204
          tunnel: [w210 w213 w216 w219 w222 w225 w228 w231 w234 w237 w240 1] -> w205
          tunnel: w203 -> [w208 w211 w214 w217 w220 w223 w226 w229 w232 w235 w238 _]
          frame "Freq" {
            n99 = Unbundle By Name(w208) -> ("FreqUnit"=w210:T37, "FreqUnitPrcs"=w209:dbl)
          }
          frame "Period" {
            n100 = Unbundle By Name(w211) -> ("PeriodUnit"=w213:enum32{"No Selection", "s", "ms", "us", "ns"}, "PeriodUnitPrcs"=w212:dbl)
          }
          frame "Ampl" {
            n101 = Unbundle By Name(w214) -> ("AmplUnit"=w216:enum32{"No Selection", "Vpp", "mVpp"}, "AmplUnitPrcs"=w215:dbl)
          }
          frame "HighL" {
            n102 = Unbundle By Name(w217) -> ("HighLUnit"=w219:enum32{"No Selection", "V", "mV"}, "HighLUnitPrcs"=w218:dbl)
          }
          frame "Offset" {
            n103 = Unbundle By Name(w220) -> ("OffsetUnit"=w222:enum32{"No Selection", "Vdc", "mVdc"}, "OffsetUnitPrcs"=w221:dbl)
          }
          frame "LowL" {
            n104 = Unbundle By Name(w223) -> ("LowLUnit"=w225:enum32{"No Selection", "V", "mV"}, "LowLUnitPrcs"=w224:dbl)
          }
          frame "Phase" {
            n105 = Unbundle By Name(w226) -> ("PhaseUnit"=w228:enum32{"°"}, "PhaseUnitPrcs"=w227:dbl)
          }
          frame "Duty" {
            n106 = Unbundle By Name(w229) -> ("DutyUnit"=w231:enum32{"%"}, "DutyUnitPrcs"=w230:dbl)
          }
          frame "Width" {
            n107 = Unbundle By Name(w232) -> ("WidthUnit"=w234:enum32{"No Selection", "s", "ms", "us", "ns"}, "WidthUnitPrcs"=w233:dbl)
          }
          frame "RisEdge" {
            n108 = Unbundle By Name(w235) -> ("RisEdgeUnit"=w237:enum32{"No Selection", "s", "ms", "us", "ns"}, "RisEdgeUnitPrcs"=w236:dbl)
          }
          frame "FallEdge" {
            n109 = Unbundle By Name(w238) -> ("FallEdgeUnit"=w240:enum32{"No Selection", "s", "ms", "us", "ns"}, "FallEdgeUnitPrcs"=w239:dbl)
          }
          frame Default {
          }
        }
        n110 = call "Get Control Ref By Label.vi"("Control Label"="Value", "Actors in"=w203) -> ("error out"=w200:errorcluster, "Control Ref"=w202:refnum<vi>, "Actors out"=w196:refnum<class "Rigol DG822 Pulse.lvclass">)  [unwired: 7 in]
        n111 = call "Value Round.vi"("error in (no error)"=w200, "UnitPrecision"=w204, "Value Ref"=w202) -> ("error out"=w199:errorcluster, "Value"=w198:dbl)  [unwired: 7 in]
        n112 = Unbundle By Name(w196) -> ("Self Enq"=w207:refnum<class "Message Enqueuer.lvclass">)
        n113 = Bundle("Value"=w198, "PeriodUnit"=w205, "FreqUnitPrecision"=w204) -> (w206:T38)  [unwired: 1 in]
        n114 = call "Send ExtCall.vi"("error in (no error)"=w199, "Val"=w206, "Tag"="ParamTags", "Message Enqueuer"=w207) -> ("error out"=w194:errorcluster)  [unwired: 4 in, 3 out]
        n115 = call "Set Concrol Value.vi"("error in (no error)"=w194, "Value"="ParamTags", "Control Label"="PulseParamDisplay", "Actors in"=w196) -> ("Actors out"=w197:refnum<class "Rigol DG822 Pulse.lvclass">)  [unwired: 6 in, 1 out]
      }
      event User Event {
        n116 = event-data() -> ("Type"=w245:u16, "Data"=w246:variant)  [unwired: 1 in]
        n117 = Type Cast(type=WaveformExtCall."Freq" ("Enum"), x=w245) -> (*(type *) &x=w244:T28)
        n118 = case shown="\"RisEdge\", \"FallEdge\"" w244 {
          selector: w244 -> [w272 w283 w299 w322 w335 _ _]
          tunnel: [w277 w292 w303 w324 w337 w340 w353] -> w248
          tunnel: w247 -> [w276 w284 w298 w321 w334 w341 w351]
          tunnel: w246 -> [w275 w282 w297 w320 w333 _ w354]
          frame "Freq", "Period" {
            n119 = Variant To Data(type=T29 {"Freq"={"Freq"=1.0, "FreqUnit"=enum."kHz", "FreqUnitPrcs"=9.0}, "Period"={"Period"=1.0, "PeriodUnit"=enum."ms", "PeriodUnitPrcs"=7.0}, "Duty"={"Duty"=50.0, "DutyUnit"=enum."%", "DutyUnitPrcs"=3.0}, "Width"={"Width"=500.0, "WidthUnit"=enum."us", "WidthUnitPrcs"=4.0}, "RisEdge"={"RisEdge"=10.0, "RisEdgeUnit"=enum."ns", "RisEdgeUnitPrcs"=1.0}, "FallEdge"={"FallEdge"=10.0, "FallEdgeUnit"=enum."ns", "FallEdgeUnitPrcs"=1.0}}, Variant=w275) -> (data=w271:T29)  [unwired: 1 in, 1 out]
            n120 = Unbundle(w271) -> ("Freq"=w270:T39, "Period"=w269:T40, "Duty"=w268:T41, "Width"=w267:T42, "RisEdge"=w265:T43, "FallEdge"=w264:T44)
            n121 = Bundle By Name(cluster=w276, "Freq"=w270, "Period"=w269, "Duty"=w268, "Width"=w267, "RisEdge"=w265, "FallEdge"=w264) -> (w250:refnum<class "Rigol DG822 Pulse.lvclass">)
            n122 = Unbundle By Name(w250) -> ("Duty/Width"=w249:bool)
            n123 = call-dynamic "Update String Values.vi"("Type"=w272, "Rigol DG822 Pulse in"=w250) -> ("error out"=w273:errorcluster, "Rigol DG822 Pulse out"=w274:refnum<class "Rigol DG822 Pulse.lvclass">)  [unwired: 8 in]
            n124 = Select(t=u16 8 ("Type"), s=w249, f=u16 7 ("Type")) -> (s? t:f=w258:u16)
            n125 = call-dynamic "Update String Values.vi"("error in (no error)"=w273, "Type"=w258, "Rigol DG822 Pulse in"=w274) -> ("error out"=w262:errorcluster, "Rigol DG822 Pulse out"=w263:refnum<class "Rigol DG822 Pulse.lvclass">)  [unwired: 7 in]
            n126 = call-dynamic "Update String Values.vi"("error in (no error)"=w262, "Type"=u16 9, "Rigol DG822 Pulse in"=w263) -> ("error out"=w254:errorcluster, "Rigol DG822 Pulse out"=w256:refnum<class "Rigol DG822 Pulse.lvclass">)  [unwired: 7 in]
            n127 = call-dynamic "Update String Values.vi"("error in (no error)"=w254, "Type"=u16 10, "Rigol DG822 Pulse in"=w256) -> ("error out"=w251:errorcluster, "Rigol DG822 Pulse out"=w255:refnum<class "Rigol DG822 Pulse.lvclass">)  [unwired: 7 in]
            n128 = call-dynamic "Send Data.vi"("error in (no error)"=w251, "Rigol DG822 Pulse in"=w255) -> ("error out"=w260:errorcluster, "Rigol DG822 Pulse out"=w261:refnum<class "Rigol DG822 Pulse.lvclass">)  [unwired: 8 in]
            n129 = call-dynamic "Reset Window.vi"("error in (no error)"=w260, "Rigol DG822 Pulse in"=w261) -> ("Rigol DG822 Pulse out"=w277:refnum<class "Rigol DG822 Pulse.lvclass">)  [unwired: 8 in, 1 out]
          }
          frame "Ampl".."LowL" {
            n130 = Variant To Data(type=T30 {"Ampl"={"Ampl"=5.0, "AmplUnit"=enum."Vpp", "AmplUnitPrcs"=4.0}, "HighL"={"HighL"=2.5, "HighLUnit"=enum."V", "HighLUnitPrcs"=4.0}, "Offset"={"Offset"=0.0, "OffsetUnit"=enum."Vdc", "OffsetUnitPrcs"=4.0}, "LowL"={"LowL"=-2.5, "LowLUnit"=enum."V", "LowLUnitPrcs"=4.0}}, Variant=w282) -> (data=w286:T30)  [unwired: 1 in, 1 out]
            n131 = Unbundle(w286) -> ("Ampl"=w287:T45, "HighL"=w290:T46, "Offset"=w289:T47, "LowL"=w288:T48)
            n132 = Bundle By Name(cluster=w284, "Ampl"=w287, "HighL"=w290, "Offset"=w289, "LowL"=w288) -> (w291:refnum<class "Rigol DG822 Pulse.lvclass">)
            n133 = call-dynamic "Update String Values.vi"("Type"=w283, "Rigol DG822 Pulse in"=w291) -> ("error out"=w280:errorcluster, "Rigol DG822 Pulse out"=w279:refnum<class "Rigol DG822 Pulse.lvclass">)  [unwired: 8 in]
            n134 = call-dynamic "Send Data.vi"("error in (no error)"=w280, "Rigol DG822 Pulse in"=w279) -> ("error out"=w278:errorcluster, "Rigol DG822 Pulse out"=w281:refnum<class "Rigol DG822 Pulse.lvclass">)  [unwired: 8 in]
            n135 = call-dynamic "Reset Window.vi"("error in (no error)"=w278, "Rigol DG822 Pulse in"=w281) -> ("Rigol DG822 Pulse out"=w292:refnum<class "Rigol DG822 Pulse.lvclass">)  [unwired: 8 in, 1 out]
          }
          frame "Phase" {
            n136 = Variant To Data(type=T31 {"Phase"=0.0, "PhaseUnit"=enum."°", "PhaseUnitPrcs"=3.0} ("Phase"), Variant=w297) -> (data=w302:T31)  [unwired: 1 in, 1 out]
            n137 = Bundle By Name(cluster=w298, "Phase"=w302) -> (w301:refnum<class "Rigol DG822 Pulse.lvclass">)
            n138 = call-dynamic "Update String Values.vi"("Type"=w299, "Rigol DG822 Pulse in"=w301) -> ("error out"=w294:errorcluster, "Rigol DG822 Pulse out"=w296:refnum<class "Rigol DG822 Pulse.lvclass">)  [unwired: 8 in]
            n139 = call-dynamic "Send Data.vi"("error in (no error)"=w294, "Rigol DG822 Pulse in"=w296) -> ("error out"=w293:errorcluster, "Rigol DG822 Pulse out"=w295:refnum<class "Rigol DG822 Pulse.lvclass">)  [unwired: 8 in]
            n140 = call-dynamic "Reset Window.vi"("error in (no error)"=w293, "Rigol DG822 Pulse in"=w295) -> ("Rigol DG822 Pulse out"=w303:refnum<class "Rigol DG822 Pulse.lvclass">)  [unwired: 8 in, 1 out]
          }
          frame "Duty", "Width" {
            n141 = Variant To Data(type=T32 {"Duty"={"Duty"=50.0, "DutyUnit"=enum."%", "DutyUnitPrcs"=3.0}, "Width"={"Width"=500.0, "WidthUnit"=enum."us", "WidthUnitPrcs"=4.0}, "FallEdge"={"FallEdge"=10.0, "FallEdgeUnit"=enum."ns", "FallEdgeUnitPrcs"=1.0}, "RisEdge"={"RisEdge"=10.0, "RisEdgeUnit"=enum."ns", "RisEdgeUnitPrcs"=1.0}}, Variant=w320) -> (data=w318:T32)  [unwired: 1 in, 1 out]
            n142 = Unbundle(w318) -> ("Duty"=w317:T41, "Width"=w316:T42, "FallEdge"=w315:T44, "RisEdge"=w314:T43)
            n143 = Bundle By Name(cluster=w321, "Duty"=w317, "Width"=w316, "RisEdge"=w315, "FallEdge"=w314) -> (w323:refnum<class "Rigol DG822 Pulse.lvclass">)
            n144 = call-dynamic "Update String Values.vi"("Type"=w322, "Rigol DG822 Pulse in"=w323) -> ("error out"=w306:errorcluster, "Rigol DG822 Pulse out"=w308:refnum<class "Rigol DG822 Pulse.lvclass">)  [unwired: 8 in]
            n145 = call-dynamic "Update String Values.vi"("error in (no error)"=w306, "Type"=u16 9, "Rigol DG822 Pulse in"=w308) -> ("error out"=w310:errorcluster, "Rigol DG822 Pulse out"=w311:refnum<class "Rigol DG822 Pulse.lvclass">)  [unwired: 7 in]
            n146 = call-dynamic "Update String Values.vi"("error in (no error)"=w310, "Type"=u16 10, "Rigol DG822 Pulse in"=w311) -> ("error out"=w304:errorcluster, "Rigol DG822 Pulse out"=w305:refnum<class "Rigol DG822 Pulse.lvclass">)  [unwired: 7 in]
            n147 = call-dynamic "Send Data.vi"("error in (no error)"=w304, "Rigol DG822 Pulse in"=w305) -> ("error out"=w312:errorcluster, "Rigol DG822 Pulse out"=w313:refnum<class "Rigol DG822 Pulse.lvclass">)  [unwired: 8 in]
            n148 = call-dynamic "Reset Window.vi"("error in (no error)"=w312, "Rigol DG822 Pulse in"=w313) -> ("Rigol DG822 Pulse out"=w324:refnum<class "Rigol DG822 Pulse.lvclass">)  [unwired: 8 in, 1 out]
          }
          frame "RisEdge", "FallEdge" {
            n149 = Variant To Data(type=T33 {"FallEdge"={"FallEdge"=10.0, "FallEdgeUnit"=enum."ns", "FallEdgeUnitPrcs"=1.0}, "RisEdge"={"RisEdge"=10.0, "RisEdgeUnit"=enum."ns", "RisEdgeUnitPrcs"=1.0}}, Variant=w333) -> (data=w332:T33)  [unwired: 1 in, 1 out]
            n150 = Unbundle(w332) -> ("FallEdge"=w326:T44, "RisEdge"=w325:T43)
            n151 = Bundle By Name(cluster=w334, "RisEdge"=w326, "FallEdge"=w325) -> (w336:refnum<class "Rigol DG822 Pulse.lvclass">)
            n152 = call-dynamic "Update String Values.vi"("Type"=w335, "Rigol DG822 Pulse in"=w336) -> ("error out"=w328:errorcluster, "Rigol DG822 Pulse out"=w329:refnum<class "Rigol DG822 Pulse.lvclass">)  [unwired: 8 in]
            n153 = call-dynamic "Send Data.vi"("error in (no error)"=w328, "Rigol DG822 Pulse in"=w329) -> ("error out"=w330:errorcluster, "Rigol DG822 Pulse out"=w331:refnum<class "Rigol DG822 Pulse.lvclass">)  [unwired: 8 in]
            n154 = call-dynamic "Reset Window.vi"("error in (no error)"=w330, "Rigol DG822 Pulse in"=w331) -> ("Rigol DG822 Pulse out"=w337:refnum<class "Rigol DG822 Pulse.lvclass">)  [unwired: 8 in, 1 out]
          }
          frame "Home", Default {
            n155 = property on="Conf Tabs" class="TabCtl (strict)"("Value"=enum32{"Pulse", "OK"}."Pulse" ("Conf Tabs")) -> (error out=w339:errorcluster)  [unwired: 2 in, 1 out]
            n156 = call-dynamic "Reset Window.vi"("error in (no error)"=w339, "Rigol DG822 Pulse in"=w341) -> ("Rigol DG822 Pulse out"=w340:refnum<class "Rigol DG822 Pulse.lvclass">)  [unwired: 8 in, 1 out]
          }
          frame "InitData" {
            n157 = Variant To Data(type=T34 {"Data"={"Freq"={"Freq"=1.0, "FreqUnit"=enum."kHz", "FreqUnitPrcs"=9.0}, "Period"={"Period"=1.0, "PeriodUnit"=enum."ms", "PeriodUnitPrcs"=7.0}, "Ampl"={"Ampl"=5.0, "AmplUnit"=enum."Vpp", "AmplUnitPrcs"=4.0}, "HighL"={"HighL"=2.5, "HighLUnit"=enum."V", "HighLUnitPrcs"=4.0}, "Offset"={"Offset"=0.0, "OffsetUnit"=enum."Vdc", "OffsetUnitPrcs"=4.0}, "LowL"={"LowL"=-2.5, "LowLUnit"=enum."V", "LowLUnitPrcs"=4.0}, "Phase"={"Phase"=0.0, "PhaseUnit"=enum."°", "PhaseUnitPrcs"=3.0}, "Duty"={"Duty"=50.0, "DutyUnit"=enum."%", "DutyUnitPrcs"=3.0}, "Width"={"Width"=500.0, "WidthUnit"=enum."us", "WidthUnitPrcs"=4.0}, "RisEdge"={"RisEdge"=10.0, "RisEdgeUnit"=enum."ns", "RisEdgeUnitPrcs"=1.0}, "FallEdge"={"FallEdge"=10.0, "FallEdgeUnit"=enum."ns", "FallEdgeUnitPrcs"=1.0}}, "F/T Ctrls"={"Freq/Period"=FALSE, "Ampl/HighL"=FALSE, "Offset/LowL"=FALSE, "Duty/Width"=FALSE}, "String Indcs"={"Freq-Period"="1.000,000,000 kHz", "Ampl-HighL"="5.000,0 Vpp", "Offset-LowL"="0.000,0 Vdc", "Phase"="0.000 °", "Duty-Width"="50.000 %", "RisEdge"="10.0 ns", "FallEdge"="10.0 ns"}} ("Params Data"), Variant=w354) -> (data=w352:T34, error out=w342:errorcluster)  [unwired: 1 in]
            n158 = Bundle By Name(cluster=w351, "Params Data"=w352) -> (w347:refnum<class "Rigol DG822 Pulse.lvclass">)
            n159 = Unbundle By Name(w347) -> ("Duty/Width"=w348:bool)
            n160 = Select(t=u16 8 ("Type"), s=w348, f=u16 7) -> (s? t:f=w343:u16)
            n161 = call-dynamic "Update String Values.vi"("error in (no error)"=w342, "Type"=w343, "Rigol DG822 Pulse in"=w347) -> ("error out"=w346:errorcluster, "Rigol DG822 Pulse out"=w349:refnum<class "Rigol DG822 Pulse.lvclass">)  [unwired: 7 in]
            n162 = call-dynamic "Init Data.vi"("error in (no error)"=w346, "Rigol DG822 Pulse in"=w349) -> ("Rigol DG822 Pulse out"=w353:refnum<class "Rigol DG822 Pulse.lvclass">)  [unwired: 8 in, 1 out]
          }
        }
      }
      event Panel Close? {
        n163 = event-data() -> ()  [unwired: 1 in, 1 out]
        n164 = flat-sequence {
          tunnel: w358 -> [w361]
          tunnel: [w361] -> w357
          tunnel: w357 -> [w363]
          tunnel: [w362] -> w356
          tunnel: [TRUE] -> w359
          tunnel: [w364] -> w355
          tunnel: w356 -> [w364]
          frame #0 {
            n165 = call "SaveBounds.vi"("SettingName"="RDG822Pulse.bounds") -> ()
          }
          frame #1 {
            n166 = call "SetClose.vi"("Actors in"=w363) -> ("Actors out"=w362:refnum<class "Rigol DG822 Pulse.lvclass">)  [unwired: 9 in, 1 out]
          }
          frame #2 {
          }
        }
        n167 = event-data("Discard?"=w359) -> ()  [unwired: 1 in, 1 out]
      }
      event User Event {
        n168 = event-data() -> ()  [unwired: 1 in, 1 out]
        n169 = flat-sequence {
          tunnel: w370 -> [w373]
          tunnel: [w372] -> w369
          tunnel: w368 -> [w372]
          tunnel: w369 -> [w374]
          tunnel: [w374] -> w367
          tunnel: [TRUE] -> w371
          tunnel: w367 -> [w375]
          tunnel: [w375] -> w366
          frame #0 {
            n170 = Unregister For Events(event registration refnum=w373) -> ()  [unwired: 1 in, 1 out]
          }
          frame #1 {
          }
          frame #2 {
          }
        }
      }
    }
  }
  n171 = call-parent "Actor Core.vi"("error in"=w10, "Actor in"=w6) -> ("error out"=w9:errorcluster, "Actor out"=w1:refnum<class "Actor.lvclass">)  [unwired: 8 in]
  n172 = flat-sequence {
    tunnel: w1 -> [w381]
    tunnel: w9 -> [w380]
    tunnel: w6 -> [w377]
    frame #0 {
      n173 = invoke class="VI" method="FP.Close"() -> ()  [unwired: 3 in, 3 out]
      n174 = call "Read Abort.vi"("Actors in"=w377) -> ("AbortEvent"=w379:refnum<notifier>)  [unwired: 10 in]
      n175 = Send Notification(notification=cluster{"Caller":string, "AnyValue":variant} {"Caller"="abort", "AnyValue"=variant}, notifier=w379) -> ()  [unwired: 1 in, 2 out]
      "Actor out" <- w381
      "error out" <- w380
    }
  }
